vi "defunct Setup acquisition.vi"(0 "Camera Parameters (important)":T4={"Exposure Time (sec)"=0.1, "EM CCD Gain"=230, "Readout Settings"={"Acquisition Mode"=enum."Single Scan", "Pixel Rate"=enum."EM CCD 1 Mhz 16 bits", "High Capacity?"=FALSE, "V Shift Speed (us/row)"=enum."3.3  (not reccommended)", "V Shift Amplitude"=enum."+2", "Preamp Gain"=enum."2.4", "Trigger Mode"=0, "Baseline offset"=0, "Baseline clamp"=FALSE}, "Image Size"={"H Bin"=1, "V Bin"=1, "Left"=1, "Top"=1, "Right"=512, "Bottom"=512}} {"Readout Settings"."Baseline offset" min=-1000 max=1000 step=100; "Readout Settings"."Trigger Mode" items=["Internal", "External"]; "EM CCD Gain" scale=1.0..300.0; "Exposure Time (sec)" scale=0.001..10.0 scale format="%#_1g"}) -> (14 "Image Size Out":T7={"H Bin"=1, "V Bin"=1, "Left"=1, "Top"=1, "Right"=512, "Bottom"=512}, 15 "Continue with acq?":bool, 16 "Glimpse file properties":T1 {"Max Space Req'd. (Gb)" format="%.2f"}, 19 "Error Out (no error)":errorcluster)   [LabVIEW 2016]
doc: "This VI sets the hardware and Glimpse parameters for acquisition from the Cascade camera. If requested, shows a live video preview to allow setting of acquisition AOI and other camera parameters. When user presses \"GO\", vi exits leaving camera setup. Intended for use as a sub-vi, interactively or non-.\n\nLimitations: does not display current temperatures"
uses:
  <vilib>/vision/Image Controls.llb/IMAQ Image.ctl
  new-h-nu-ixon/Laser type.ctt
  Camera/camera globals.vi
  Camera/Glimpse file parameters.ctt
  new-h-nu-ixon/Emission filters.ctl
  ixon ultra 897/HAL camera parameters important.ctt
  ixon ultra 897/andor acquisition mode.ctl
  ixon ultra 897/ixon readout settings.ctl
panel:
  in  "Set to AOI":bool
  in  "Set to 512 x 300":bool
  in  "Set to 512 x 512":bool
  out "Actual Exposure Time (sec)":sgl format="%.4f"
  in  "Preview Shutters":T2[](array[typedef])
  in  "Preview emission filter":T3
  in  "Number of preview windows":i32=1
  in  "Go? (F)":bool
  in  "Quit":bool
  in  "Preview?":bool
  # "Parameters for non-interactive use"
  # "Camera: Andor iXon"
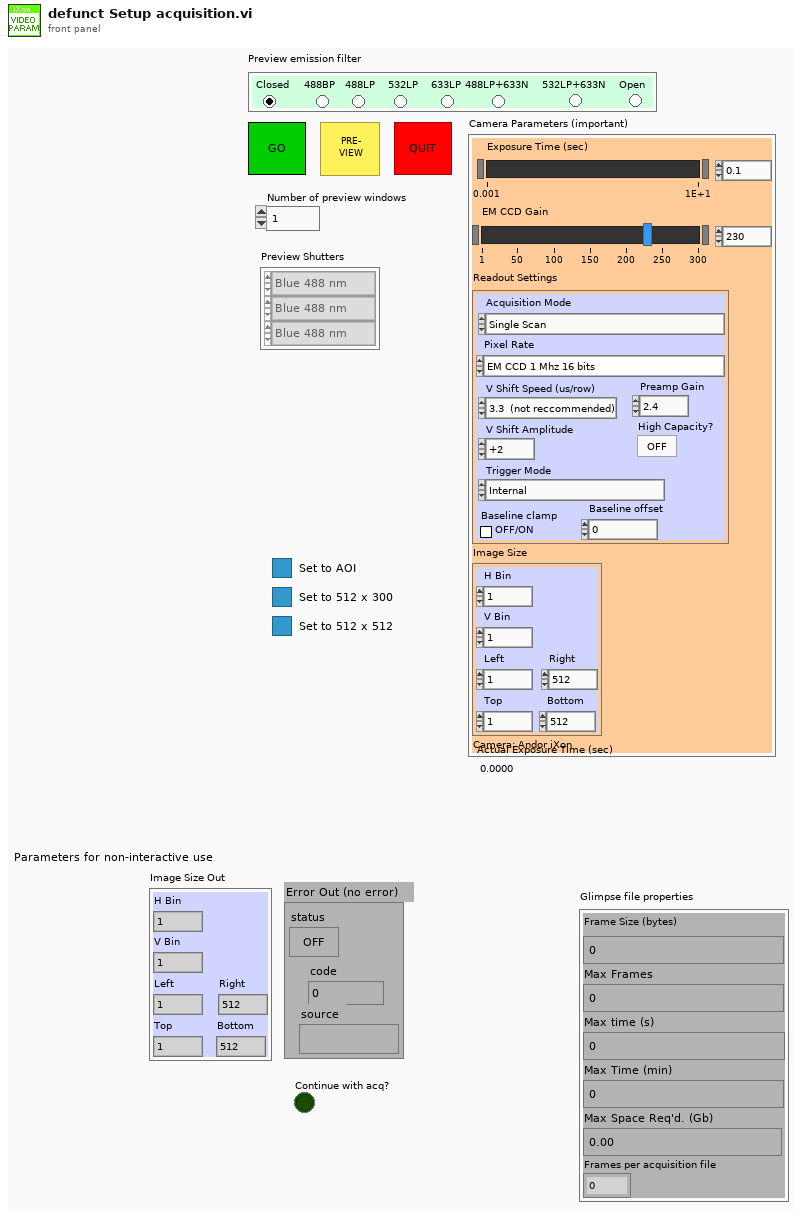
[diagram p1: front panel]
types:
  T1 = typedef "Glimpse file parameters.ctt" = cluster{"Frame Size (bytes)":u32, "Max Frames":u32, "Max time (s)":u32, "Max Time (min)":u32, "Max Space Req'd. (Gb)":dbl, "Frames per acquisition file":u32}
  T2 = typedef "Laser type.ctt" = enum16{"Blue 488 nm", "Green 532 nm", "Red 633 nm", "IR 780"}
  T3 = typedef "Emission filters.ctl" = enum32{" Closed ", " 488BP ", "488LP", "  532LP ", "633LP", "488LP+633N", "532LP+633N", "Open"}
  T4 = typedef "HAL camera parameters important.ctt" = cluster{"Exposure Time (sec)":sgl, "EM CCD Gain":u16, "Readout Settings":T5, "Image Size":cluster{"H Bin":i32, "V Bin":i32, "Left":i32, "Top":i32, "Right":i32, "Bottom":i32}}
  T5 = typedef "ixon readout settings.ctl" = cluster{"Acquisition Mode":T6, "Pixel Rate":enum16{"EM CCD 10 Mhz 14 bits", "EM CCD 5 Mhz 14 bits", "EM CCD 3 Mhz 14 bits", "EM CCD 1 Mhz 16 bits", "Standard CCD 3 Mhz 14 bits", "Standard CCD 1 Mhz 16 bits"}, "High Capacity?":bool, "V Shift Speed (us/row)":enum16{"0.9 (not reccommended)", "1.7  (not reccommended)", "3.3  (not reccommended)", "6.5", "12.9"}, "V Shift Amplitude":enum16{"normal", "+1", "+2", "+3", "+4"}, "Preamp Gain":enum16{"1.0", "2.4", "5.0"}, "Trigger Mode":u32, "Baseline offset":i16, "Baseline clamp":bool}
  T6 = typedef "andor acquisition mode.ctl" = enum16{"(do not use)", "Single Scan", "Accumulate", "Kinetics", "Fast Kinetics", "Kinetics Run till Abort", "Frame Transfer", "Frame Transfer Run till Abort", "(do not use) ", "Time Delayed Integration"}
  T7 = cluster{"H Bin":i32, "V Bin":i32, "Left":i32, "Top":i32, "Right":i32, "Bottom":i32}
  T8 = typedef "IMAQ Image.ctl" = refnum<image>
  T9 = typedef "ROI Descriptor" = cluster{"Global Rectangle":i32[], "Contours":cluster{"ID":enum32{"External", "Internal"}, "Type":u32, "Coordinates":i32[]}[]}
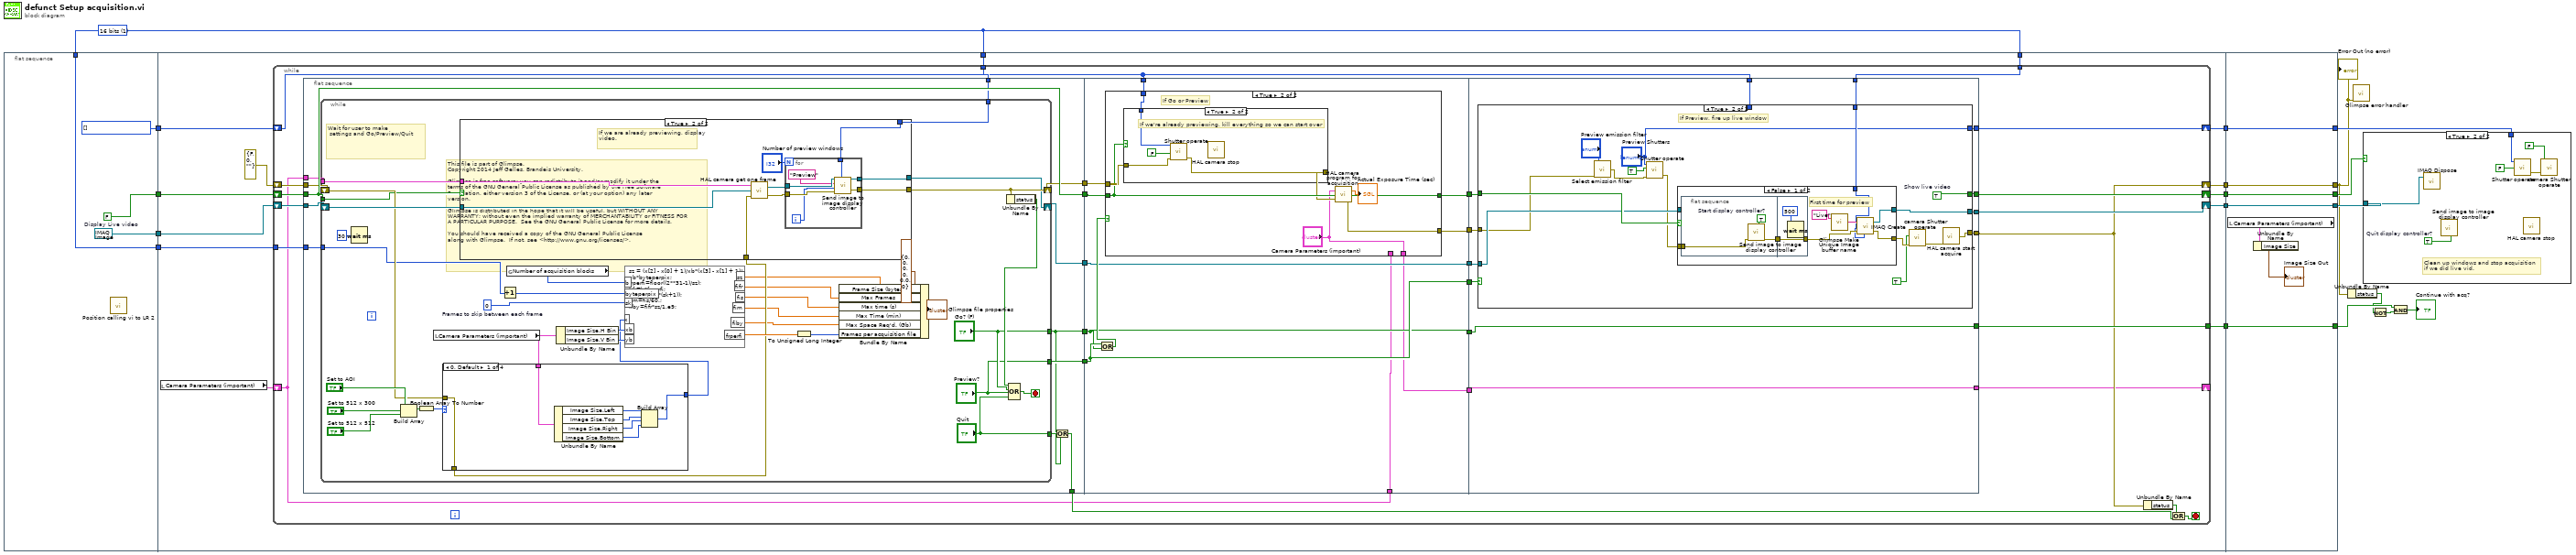
[diagram p0: block diagram]
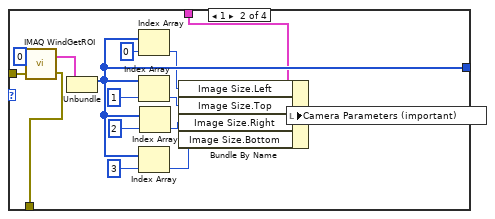
[diagram p3: hidden frame]
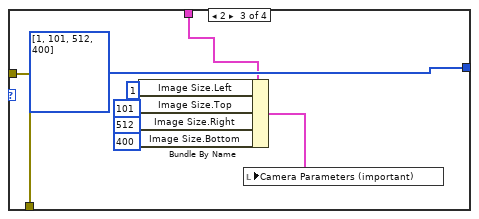
[diagram p4: hidden frame]
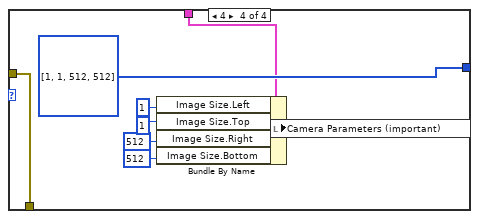
[diagram p5: hidden frame]
diagram:
  w11 = u32 1 items=["8 bits", "16 bits", "Float", "Complex", "RGB", "HSL"] ("Image Type")
  # "This file is part of Glimpse. \nCopyright 2014 Jeff Gelles, Brandeis University.    \n\nGlimpse is free software: you can redistribute it and/or modify it under the \nterms of the GNU General Public License as published by the Free Software \nFoundation, either version 3 of the License, or (at your option) any later \nversion.\n\nGlimpse is distributed in the hope that it will be useful, but WITHOUT ANY \nWARRANTY; without even the implied warranty of MERCHANTABILITY or FITNESS FOR \nA PARTICULAR PURPOSE.  See the GNU General Public License for more details.\n\nYou should have received a copy of the GNU General Public License\nalong with Glimpse.  If not, see <http://www.gnu.org/licenses/>."
  n1 = flat-sequence {
    tunnel: [w22] -> w16
    tunnel: [T8 refnum ("New Image")] -> w14
    tunnel: w11 -> [w19]
    tunnel: [w20] -> w10
    tunnel: [w19] -> w8
    tunnel: w16 -> [w35]
    tunnel: w14 -> [w31]
    tunnel: w11 -> [w29]
    tunnel: w11 -> [w28]
    tunnel: w10 -> [w27]
    tunnel: w8 -> [w25]
    tunnel: [w34] -> w7
    tunnel: [w33] -> w6
    tunnel: [w32] -> w5
    tunnel: [w30] -> w4
    tunnel: [w26] -> w3
    tunnel: [w242] -> w9
    tunnel: [w243] -> w13
    tunnel: [w244] -> w17
    tunnel: [w245] -> w2
    tunnel: [w246] -> w18
    tunnel: w7 -> [w246]
    tunnel: w6 -> [w245]
    tunnel: w5 -> [w244]
    tunnel: w4 -> [w243]
    tunnel: w3 -> [w242]
    frame #0 {
      w20 = T2[] [] items=["Blue 488 nm", "Green 532 nm", "Red 633 nm", "IR 780"] ("Preview Shutters")
      w22 = FALSE  # Display Live video
      n2 = call "Position calling vi to LR 2.vi"() -> ()  [unwired: 2 in, 4 out]
    }
    frame #1 {
      n3 = local read "Camera Parameters (important)"() -> (w23:T4)
      n4 = while {
        shift-right: [w61] -> w34
        shift-left: w35 -> [w63]
        shift-right: [w60] -> w30
        shift-left: w31 -> [w50]
        shift-right: [w39] -> w33
        shift-left: errorcluster {"status"=FALSE, "code"=0, "source"=""} ("error out") -> [w62]
        tunnel: [w59] -> w32
        tunnel: w29 -> [w44]
        tunnel: w28 -> [w43]
        shift-right: [w42] -> w26
        shift-left: w27 -> [w41]
        tunnel: w25 -> [w40]
        shift-right: [w37] -> _
        shift-left: w23 -> [w36]
        stop <- w49 stop-if-true
        n5 = flat-sequence {
          tunnel: w63 -> [w75]
          tunnel: [w75] -> w58
          tunnel: w50 -> [w74]
          tunnel: w62 -> [w73]
          tunnel: [w72] -> w57
          tunnel: [w69] -> w56
          tunnel: [w71] -> w55
          tunnel: [w68] -> w47
          tunnel: [w67] -> w46
          tunnel: w44 -> [w66]
          tunnel: w40 -> [w65]
          tunnel: w36 -> [w64]
          tunnel: w58 -> [w175]
          tunnel: [w172] -> w54
          tunnel: [w178] -> w53
          tunnel: w57 -> [w177]
          tunnel: w56 -> [w172]
          tunnel: w55 -> [w176]
          tunnel: [w176] -> w52
          tunnel: [w173] -> w51
          tunnel: w46 -> [w171]
          tunnel: [w171] -> w45
          tunnel: w41 -> [w170]
          tunnel: [w169] -> w38
          tunnel: w36 -> [w168]
          tunnel: w51 -> [w203]
          tunnel: [w202] -> w61
          tunnel: [w201] -> w60
          tunnel: [w200] -> w39
          tunnel: [w199] -> w59
          tunnel: w54 -> [w199]
          tunnel: w53 -> [w204]
          tunnel: w52 -> [w205]
          tunnel: w45 -> [w198]
          tunnel: w43 -> [w197]
          tunnel: [w196] -> w42
          tunnel: w41 -> [w195]
          tunnel: w38 -> [w194]
          tunnel: [w194] -> w37
          frame #0 {
            n6 = while {
              shift-left: w73 -> [w105]
              shift-right: [w100] -> w72
              tunnel: ["Go? (F)"] -> w69
              tunnel: w75 -> [w102]
              tunnel: ["Preview?"] -> w71
              tunnel: ["Quit"] -> w70
              shift-right: [w98] -> w67
              shift-left: w74 -> [w106]
              tunnel: w66 -> [w97]
              tunnel: w65 -> [w95]
              tunnel: w64 -> [w86]
              stop <- w87 stop-if-true
              w101 = u16 0  # Frames to skip between each frame
              # "Wait for user to make\n settings and Go/Preview/Quit"
              n7 = Wait (ms)(milliseconds to wait=u32 30) -> ()  [unwired: 1 out]
              n8 = Build Array("Set to AOI", "Set to 512 x 300", "Set to 512 x 512") -> (w111:bool[])
              n9 = Boolean Array To Number(Boolean array=w111) -> (number=w107:u32)
              n10 = local read "Camera Parameters (important)"() -> (w85:T4)
              n11 = case shown="0, Default" w107 {
                tunnel: w105 -> [w136 w151 w159 w167]
                tunnel: [w130 w144 i32[] [1, 101, 512, 400] ("Global Rectangle") i32[] [1, 1, 512, 512] ("Global Rectangle")] -> w92
                tunnel: [w136 w149 w159 w167] -> w99
                tunnel: w85 -> [w131 w137 w152 w160]
                frame 0, Default {
                  n12 = Unbundle By Name(w131) -> ("Image Size.Left"=w132:i32, "Image Size.Top"=w133:i32, "Image Size.Right"=w134:i32, "Image Size.Bottom"=w135:i32)
                  n13 = Build Array(w132, w133, w134, w135) -> (w130:i32[])
                }
                frame 1 {
                  n14 = call "IMAQ WindGetROI"("Window Number (0...15)"=0, "error in (no error)"=w151) -> ("ROI Descriptor"=w150:T9, "error out"=w149:errorcluster)  [unwired: 3 out]
                  n15 = Unbundle(w150) -> ("Global Rectangle"=w144:i32[])  [unwired: 1 out]
                  n16 = Index Array(array=w144, index=0) -> (element=w142:i32)
                  n17 = Index Array(array=w144, index=1) -> (element=w141:i32)
                  n18 = Index Array(array=w144, index=3) -> (element=w139:i32)
                  n19 = Index Array(array=w144, index=2) -> (element=w140:i32)
                  n20 = Bundle By Name(cluster=w137, "Image Size.Left"=w142, "Image Size.Top"=w141, "Image Size.Right"=w140, "Image Size.Bottom"=w139) -> (w143:T4)
                  n21 = local write "Camera Parameters (important)"(w143) -> ()
                }
                frame 2 {
                  n22 = Bundle By Name(cluster=w152, "Image Size.Left"=1 ("Left"), "Image Size.Top"=101 ("Top"), "Image Size.Right"=512 ("Right"), "Image Size.Bottom"=400 ("Bottom")) -> (w156:T4)
                  n23 = local write "Camera Parameters (important)"(w156) -> ()
                }
                frame 4 {
                  n24 = Bundle By Name(cluster=w160, "Image Size.Left"=1 ("Left"), "Image Size.Top"=1 ("Top"), "Image Size.Right"=512 ("Right"), "Image Size.Bottom"=512 ("Bottom")) -> (w164:T4)
                  n25 = local write "Camera Parameters (important)"(w164) -> ()
                }
              }
              n26 = case shown="True" w102 {
                tunnel: w106 -> [w112 w121]
                tunnel: [w113 w119] -> w100
                tunnel: w99 -> [w113 w122]
                tunnel: [w112 w120] -> w98
                tunnel: w97 -> [_ w115]
                tunnel: w86 -> [_ w114]
                frame False {
                }
                frame True {
                  # "If we are already previewing, display video."
                  n27 = call "HAL camera get one frame.vi"("error in"=w122, "New Image"=w121, "Camera Parameters (important)"=w114) -> ("error out"=w118:errorcluster, "Image Out"=w116:T8)
                  n28 = for {
                    N: "Number of preview windows" -> [_]
                    tunnel: [w129] -> w120
                    tunnel: [w128] -> w119
                    tunnel: w118 -> [w127]
                    tunnel: w116 -> [w126]
                    tunnel: w115 -> [w123]
                    i -> [w124]
                    n29 = call "Send image to image display controller.vi"("Image"=w126, "Window Title"="Preview" ("Window Title\n(Window only)"), "Window Number"=w124, "error in"=w127, "Image Type"=w123) -> ("Image Out"=w129:T8, "error out"=w128:errorcluster)  [unwired: 2 in, 2 out]
                  }
                }
              }
              n30 = Increment(x=w95) -> (x+1=w96:u32)
              n31 = global read "camera globals.vi" "Number of acquisition blocks"() -> (w84:i8)
              n32 = Unbundle By Name(w85) -> ("Image Size.H Bin"=w94:i32, "Image Size.V Bin"=w93:i32)
              n33 = formula code="sz = (x[2] - x[0] + 1)/xb*(x[3] - x[1] + 1)/yb*byteperpix;\nfrperfi=floor((2**31-1)/sz);\nfifr=b*frperfi;\nfis=fifr/(30*(sk+1));\nfim=fis/60.;\nfiby=fifr*sz/1.e9;"("x"=w92, "b"=w84, "sk"=w101, "xb"=w94, "yb"=w93, "byteperpix"=w96) -> ("sz"=w77:dbl, "fifr"=w76:dbl, "fis"=w78:dbl, "fim"=w79:dbl, "fiby"=w80:dbl, "frperfi"=w103:dbl)
              n34 = To Unsigned Long Integer(number=w103) -> (unsigned 32bit integer=w81:u32)
              n35 = Bundle By Name(cluster=T1 {"Frame Size (bytes)"=0, "Max Frames"=0, "Max time (s)"=0, "Max Time (min)"=0, "Max Space Req'd. (Gb)"=0.0, "Frames per acquisition file"=0} ("Glimpse file properties"), "Frame Size (bytes)"=w77, "Max Frames"=w76, "Max time (s)"=w78, "Max Time (min)"=w79, "Max Space Req'd. (Gb)"=w80, "Frames per acquisition file"=w81) -> (→"Glimpse file properties":T1)
              n36 = Unbundle By Name(w100) -> ("status"=w91:bool)
              n37 = Compound Arithmetic op=OR(w91, "Go? (F)", "Preview?", "Quit") -> (w87:bool)
            }
            n38 = Or(x=w69, y=w70) -> (x .or. y?=w68:bool)
          }
          frame #1 {
            n39 = Or(x=w176, y=w172) -> (x .or. y?=w174:bool)
            n40 = case shown="True" w174 {
              tunnel: [w181 w183] -> w178
              tunnel: w177 -> [w181 w187]
              tunnel: w175 -> [w180 w188]
              tunnel: [w180 w188] -> w173
              tunnel: w170 -> [_ w186]
              tunnel: [w179 "Camera Parameters (important)"] -> w169
              tunnel: w168 -> [w179 _]
              frame False {
              }
              frame True {
                # "If Go or Preview"
                n41 = case shown="True" w188 {
                  tunnel: w187 -> [w189 w190]
                  tunnel: [w189 w192] -> w185
                  tunnel: w186 -> [_ w191]
                  frame False {
                  }
                  frame True {
                    # "If we're already previewing, kill everything so we can start over"
                    n42 = call "Shutter operate.vi"("Shutters"=w191, 2:FALSE, "error in"=w190) -> ("error out"=w192:errorcluster)  [unwired: 5 out]
                    n43 = call "HAL camera stop.vi"() -> ()  [unwired: 1 out]
                  }
                }
                n44 = call "HAL camera program for acquisition.vi"("error in"=w185, "Camera Parameters (important)"="Camera Parameters (important)") -> ("error out"=w183:errorcluster, "Actual Exposure Time (sec)"=→"Actual Exposure Time (sec)":sgl)
              }
            }
          }
          frame #2 {
            n45 = case shown="True" w205 {
              tunnel: w204 -> [w208 w210]
              tunnel: [w209 w224] -> w202
              tunnel: w203 -> [w209 w222]
              tunnel: [w207 w223] -> w201
              tunnel: [w208 w215] -> w200
              tunnel: w198 -> [w207 w221]
              tunnel: w197 -> [_ w220]
              tunnel: [w206 "Preview Shutters"] -> w196
              tunnel: w195 -> [w206 _]
              frame False {
              }
              frame True {
                w224 = TRUE  # Show live video
                # "If Preview, fire up live window"
                n46 = call "Select emission filter.vi"("error in"=w210, "Emission filter"="Preview emission filter") -> ("error out"=w211:errorcluster)
                n47 = call "Shutter operate.vi"("Shutters"="Preview Shutters", 2:TRUE, "error in"=w211) -> ("error out"=w218:errorcluster)  [unwired: 5 out]
                n48 = case shown="False" w222 {
                  tunnel: [w232 w238] -> w216
                  tunnel: [w229 w239] -> w223
                  tunnel: w221 -> [_ w239]
                  tunnel: w220 -> [w225 _]
                  tunnel: w218 -> [w228 w238]
                  frame False {
                    # "First time for preview"
                    n49 = flat-sequence {
                      tunnel: w228 -> [w234]
                      tunnel: [w233] -> w226
                      tunnel: [w237] -> w227
                      tunnel: w226 -> [w237]
                      frame #0 {
                        w235 = TRUE  # Start display controller?
                        n50 = call "Send image to image display controller.vi"("error in"=w234, "Start display controller?"=w235) -> ("error out"=w233:errorcluster)  [unwired: 5 in, 3 out]
                      }
                      frame #1 {
                        n51 = Wait (ms)(milliseconds to wait=u32 500) -> ()  [unwired: 1 out]
                      }
                    }
                    n52 = call "Glimpse Make Unique Image buffer name.vi"("Buffer  base name"="Live" ("Image Name")) -> ("Image Name"=w230:string)  [unwired: 1 in]
                    n53 = call "IMAQ Create"("Image Name"=w230, "Image Type"=w225, "error in (no error)"=w227) -> ("New Image"=w229:T8, "error out"=w232:errorcluster)  [unwired: 1 in, 1 out]
                  }
                  frame True {
                  }
                }
                n54 = call "camera Shutter operate.vi"("Open?"=TRUE, "error in"=w216) -> ("error out"=w214:errorcluster)  [unwired: 6 out]
                n55 = call "HAL camera start acquire.vi"("error in"=w214) -> ("error out"=w215:errorcluster)
              }
            }
          }
        }
        n56 = Unbundle By Name(w39) -> ("status"=w48:bool)
        n57 = Or(x=w48, y=w47) -> (x .or. y?=w49:bool)
      }
    }
    frame #2 {
      n58 = local read "Camera Parameters (important)"() -> (w241:T4)
      n59 = Unbundle By Name(w241) -> ("Image Size"=→"Image Size Out":T7)
    }
  }
  n60 = Unbundle By Name(w2) -> ("status"=w12:bool)
  n61 = call "Glimpse error handler.vi"("error in"=w2) -> ()  [unwired: 1 in, 6 out]
  n62 = case shown="True" w18 {
    tunnel: w13 -> [_ w252]
    tunnel: w9 -> [_ w250]
    frame False {
    }
    frame True {
      w249 = TRUE  # Quit display controller?
      # "Clean up windows and stop acquisition\nif we did live vid."
      n63 = call "IMAQ Dispose"("Image"=w252) -> ()  [unwired: 2 in, 4 out]
      n64 = call "Send image to image display controller.vi"("Quit display controller?"=w249) -> ()  [unwired: 6 in, 4 out]
      n65 = call "Shutter operate.vi"("Shutters"=w250, 2:FALSE) -> ("error out"=w247:errorcluster)  [unwired: 1 in, 5 out]
      n66 = call "HAL camera stop.vi"() -> ()  [unwired: 1 out]
      n67 = call "camera Shutter operate.vi"("Open?"=FALSE, "error in"=w247) -> ()  [unwired: 7 out]
    }
  }
  n68 = Not(x=w12) -> (.not. x?=w15:bool)
  n69 = And(x=w17, y=w15) -> (x .and. y?=→"Continue with acq?":bool)
  "Error Out (no error)" <- w2
